vi "Launch.vi"() -> ()   [LabVIEW 2015]
uses:
  Main/Load App.vi
  Main/Main.lvclass
panel:
  out "Current Action":string caption="Current Action:"
  out "Waiting Lights":T1
  out "Application Name":string
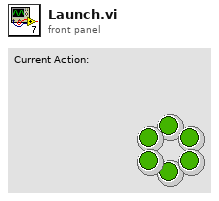
[diagram p1: front panel]
types:
  T1 = cluster{"wait 1":bool, "wait 2":bool, "wait 3":bool, "wait 4":bool, "wait 5":bool, "wait 6":bool}
  T2 = cluster{"[0]":bool, "[1]":bool, "[2]":bool, "[3]":bool, "[4]":bool, "[5]":bool}
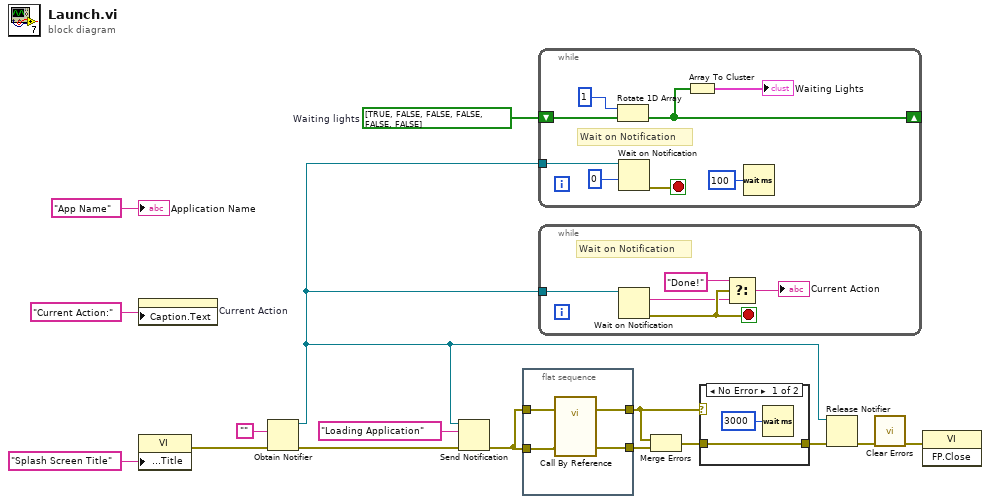
[diagram p0: block diagram]
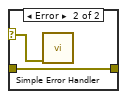
[diagram p2: hidden frame]
diagram:
  w5 = bool[] [TRUE, FALSE, FALSE, FALSE, FALSE, FALSE]  # Waiting lights
  n1 = property on="Current Action" class="Str"("Caption.Text"="Current Action:" ("Window Title")) -> ()  [unwired: 2 in, 2 out]
  n2 = property on="Property Node" class="VI"("Front Panel.Title"="Splash Screen Title" ("Window Title")) -> (error out=w1:errorcluster)  [unwired: 2 in, 1 out]
  n3 = Obtain Notifier(notification data type="" ("Empty String Constant"), error in (no error)=w1) -> (notifier out=w15:refnum<notifier>, error out=w7:errorcluster)  [unwired: 2 in, 1 out]
  n4 = Send Notification(notification="Loading Application", notifier=w15, error in (no error)=w7) -> (error out=w16:errorcluster)  [unwired: 1 out]
  n5 = flat-sequence {
    tunnel: [w19] -> w13
    tunnel: [w17] -> w14
    tunnel: w16 -> [w20]
    tunnel: w16 -> [w18]
    frame #0 {
      n6 = call-by-ref "?"(error in=w20, "error in"=w18) -> (error out=w19:errorcluster, 0:"error out"=w17:errorcluster)  [unwired: 11 in, 1 out]
    }
  }
  n7 = while {
    shift-right: [w22] -> _
    shift-left: w5 -> [w24]
    tunnel: w15 -> [w26]
    stop <- w28 stop-if-true
    # "Wait on Notification"
    n8 = Rotate 1D Array(1:w24, 2:1 ("n")) -> (0:w22:bool[])
    n9 = Wait on Notification(notifier=w26, timeout in ms (-1)=0) -> (error out=w28:errorcluster)  [unwired: 2 in, 3 out]
    n10 = Array To Cluster(array=w22) -> (cluster=→"Waiting Lights":T2)
    n11 = Wait (ms)(milliseconds to wait=u32 100) -> ()  [unwired: 1 out]
  }
  n12 = while {
    tunnel: w15 -> [w33]
    stop <- w32 stop-if-true
    # "Wait on Notification"
    n13 = Wait on Notification(notifier=w33) -> (notification=w30:string, error out=w32:errorcluster)  [unwired: 3 in, 2 out]
    n14 = Select(t="Done!" ("notification"), s=w32, f=w30) -> (s? t:f=→"Current Action":string)
  }
  n15 = Merge Errors(w13, w14) -> (w9:errorcluster)
  n16 = case shown="No Error" w13 {
    tunnel: [w35 w36] -> w8
    tunnel: w9 -> [w35 w36]
    selector: w13 -> [_ w37]
    frame No Error {
      n17 = Wait (ms)(milliseconds to wait=u32 3000) -> ()  [unwired: 1 out]
    }
    frame Error {
      n18 = call <vilib>:"Simple Error Handler.vi"("error in (no error)"=w37) -> ()  [unwired: 4 in, 5 out]
    }
  }
  n19 = Release Notifier(notifier=w15, error in (no error)=w8) -> (error out=w2:errorcluster)  [unwired: 1 in, 2 out]
  n20 = call <vilib>:"Clear Errors.vi"("error in (no error)"=w2) -> ("error out"=w6:errorcluster)  [unwired: 5 in, 1 out]
  n21 = invoke on="Invoke Node" class="VI" method="FP.Close"(error in=w6) -> ()  [unwired: 2 in, 3 out]
  "Application Name" <- "App Name" ("Unlocalized")
